vi "FindFWHM.vi"(0 "X":dbl[](array[numeric]), 1 "Y":dbl[](array[numeric])) -> (2 "FWHM":dbl format="%.2g", 3 "measurement info":T1 caption="测量信息" {"ref levels"."ref units" items=["绝对", "相对"]; "ref levels"."high ref level" format="%.2p"; "ref levels"."low ref level" format="%.2p"; "ref levels"."mid ref level" format="%.2p"; "pulse center" format="%.2p"}, 4 "center":dbl)   [LabVIEW 2018]
uses:
  <vilib>/measure/mascope.llb/Pulse Measurements 1 chan.vi
  <vilib>/measure/NI_MAPro.lvlib
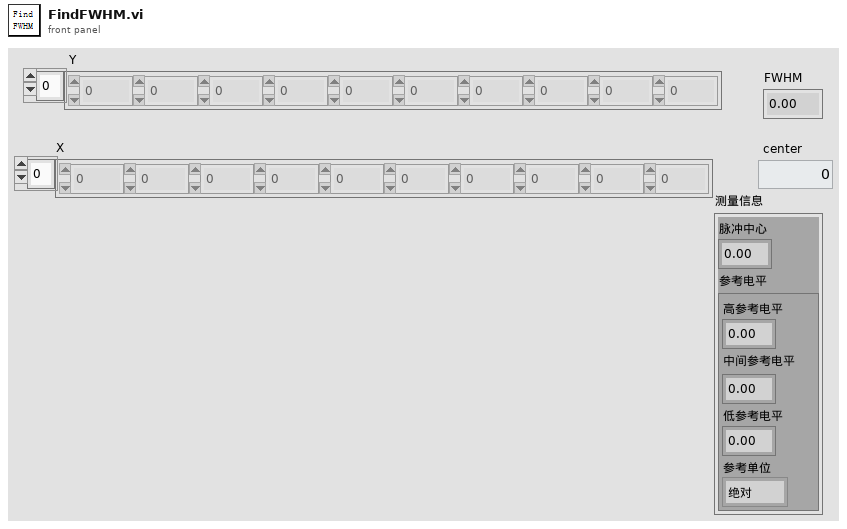
[diagram p1: front panel]
types:
  T1 = cluster{"pulse center":dbl, "ref levels":cluster{"high ref level":dbl, "mid ref level":dbl, "low ref level":dbl, "ref units":u16}}
  T2 = cluster{"method":enum32{"histogram", "peak", "auto select"}, "histogram size":i32, "histogram method":enum16{"mode"}, "reserved":dbl}
  T3 = cluster{"high ref level":dbl, "mid ref level":dbl, "low ref level":dbl, "ref units":u16}
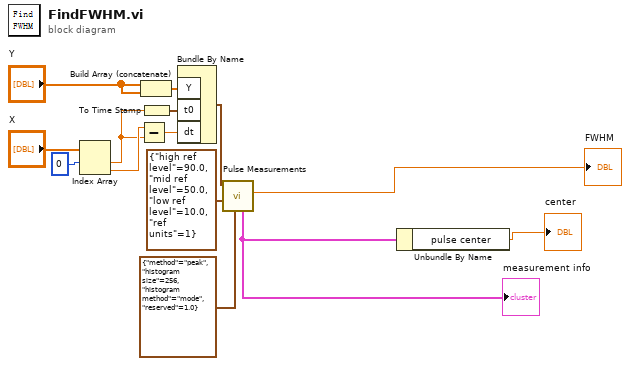
[diagram p0: block diagram]
diagram:
  n1 = Index Array(array="X", index #1=0 ("索引")) -> (element #1=w6:dbl, element #2=w7:dbl)  [unwired: 1 in]
  n2 = Subtract(x=w7, y=w6) -> (x-y=w12:dbl)
  n3 = Build Array (concatenate)("Y", "Y") -> (w9:dbl[])
  n4 = To Time Stamp(1:w6) -> (0:w13:timestamp)
  n5 = Bundle By Name("Y"=w9, "t0"=w13, "dt"=w12) -> (w11:waveform(dbl))  [unwired: 1 in]
  n6 = call-poly <vilib>:"Pulse Measurements.vi"("percent level settings"=T2 {"method"=enum."peak", "histogram size"=256, "histogram method"=enum."mode", "reserved"=1.0}, "reference levels"=T3 {"high ref level"=90.0, "mid ref level"=50.0, "low ref level"=10.0, "ref units"=1}, "signal in"=w11) -> ("pulse duration"=→"FWHM":dbl, "measurement info"=w2:T1)  [unwired: 4 in, 3 out]
  "measurement info" <- w2
  n7 = Unbundle By Name(w2) -> ("pulse center"=→"center":dbl)
